vi "CreateVisionCluster.vi"() -> (3 "Cluster":T1)   [LabVIEW 2015]
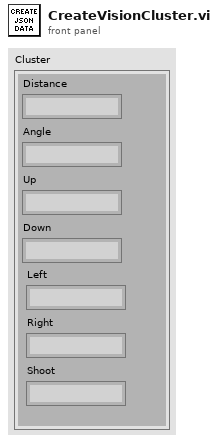
[diagram p1: front panel]
types:
  T1 = cluster{"Distance":string, "Angle":string, "Up":string, "Down":string, "Left":string, "Right":string, "Shoot":string}
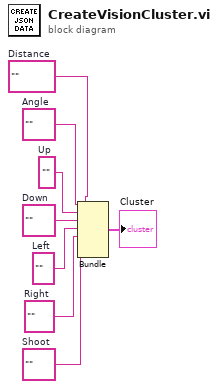
[diagram p0: block diagram]
diagram:
  w2 = ""  # Shoot
  w3 = ""  # Right
  w6 = ""  # Up
  w5 = ""  # Down
  w4 = ""  # Left
  w7 = ""  # Angle
  w8 = ""  # Distance
  n1 = Bundle("Distance"=w8, "Angle"=w7, "Up"=w6, "Down"=w5, "Left"=w4, "Right"=w3, "Shoot"=w2) -> (→"Cluster":T1)  [unwired: 1 in]
